vi "Update Messages Access Scope.vi"(8 "error in (no error)":errorcluster, 9 "scope":T1(ring)=enum."private", 10 "message parameters":T2[](array[typedef]), 11 "library in":refnum<vi>) -> (0 "error out":errorcluster, 3 "library out":refnum<vi>)   [LabVIEW 2019, in "gRPC Template Creation Utility.lvlib"]
uses:
  gRPC Template Creation Utility.lvlib
  TypeDefs/Message Metadata (Scripting).ctl
  TypeDefs/Message Element Metadata (Scripting).ctl
  TypeDefs/Message Element Type.ctl
  Oneof API/OneOf Constants/OneOfConstantsEnum.ctl
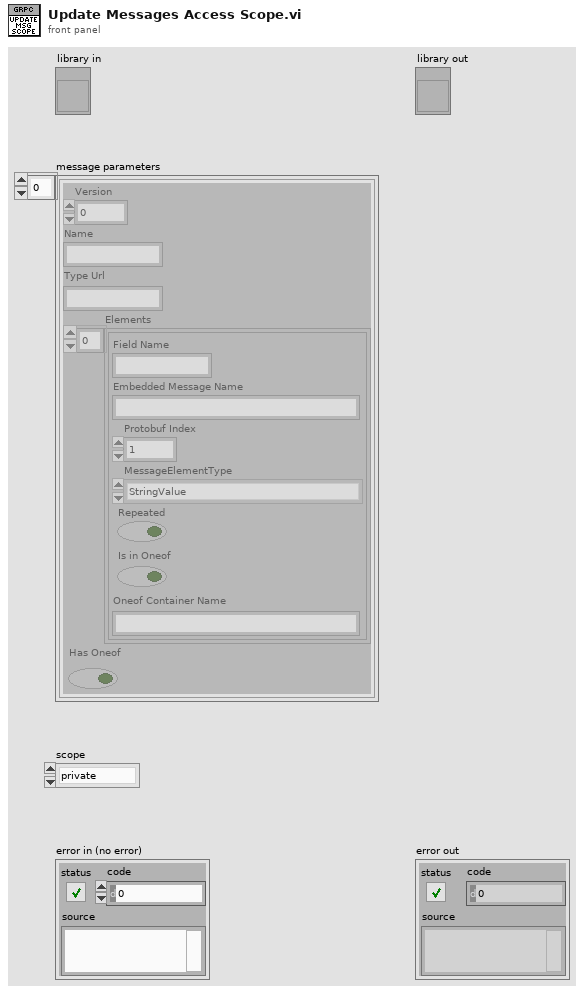
[diagram p1: front panel]
types:
  T1 = enum32{"invalid scope", "public", "private", "protected", "community"}
  T2 = typedef "gRPC Template Creation Utility.lvlib/Message Metadata (Scripting).ctl" = cluster{"Version":i32, "Name":string, "Type Url":string, "Elements":T3[], "Has Oneof":bool}
  T3 = typedef "gRPC Template Creation Utility.lvlib/Message Element Metadata (Scripting).ctl" = cluster{"Field Name":string, "Embedded Message Name":string, "Protobuf Index":i32, "MessageElementType":T4, "Repeated":bool, "Is in Oneof":bool, "Oneof Container Name":string}
  T4 = typedef "gRPC Template Creation Utility.lvlib/Message Element Type.ctl" = enum32{"Int32Value", "FloatValue", "DoubleValue", "BoolValue", "StringValue", "MessageValue", "Int64Value", "UInt32Value", "UInt64Value", "EnumValue", "Bytes", "Fixed64", "Fixed32", "SFixed64", "SFixed32", "SInt64", "SInt32"}
  T5 = typedef "gRPC Template Creation Utility.lvlib/OneOfConstantsEnum.ctl" = enum16{"FlatToRichVIPrefix", "RichToFlatVIPrefix", "FlatTypeDefSuffix"}
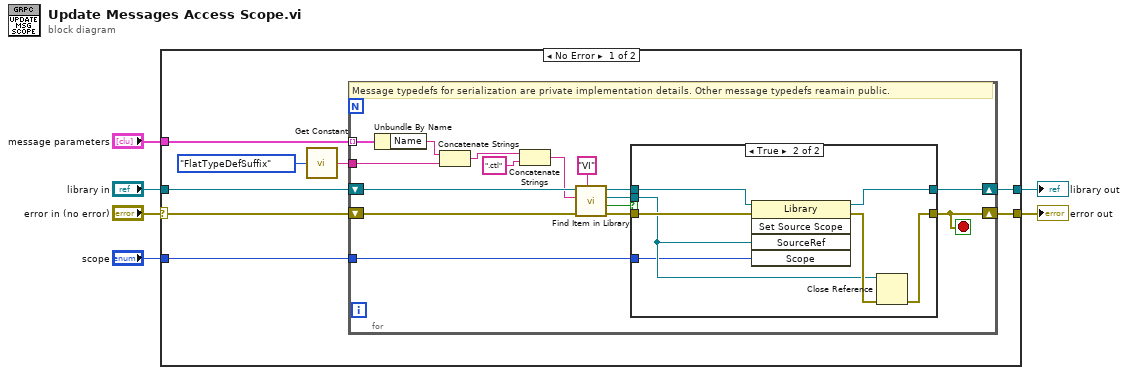
[diagram p0: block diagram]
diagram:
  n1 = case shown="No Error" "error in (no error)" {
    selector: "error in (no error)" -> [w10 w40]
    tunnel: "message parameters" -> [w14 _]
    tunnel: [w13 w41] -> w5
    tunnel: [w12 w40] -> w4
    tunnel: "library in" -> [w11 w41]
    tunnel: "scope" -> [w9 _]
    frame No Error {
      n2 = call "Get Constant.vi"("Selection"=OneOfConstantsEnum."FlatTypeDefSuffix") -> ("String"=w8:string)
      n3 = for {
        shift-right: [w18] -> w13
        shift-left: w11 -> [w26]
        shift-right: [w17] -> w12
        shift-left: w10 -> [w19]
        tunnel: w14 -> [w30] mode=indexing
        tunnel: w9 -> [w16]
        tunnel: w8 -> [w15]
        stop <- w17 stop-if-true
        # "Message typedefs for serialization are private implementation details. Other message typedefs reamain public."
        n4 = Unbundle By Name(w30) -> ("Name"=w27:string)
        n5 = Concatenate Strings(w27, w15) -> (w28:string)
        n6 = Concatenate Strings(w28, ".ctl" ("string")) -> (w25:string)
        n7 = call "Find Item in Library.vi"("Item Type"="VI" ("Type"), "error in (no error)"=w19, "Item Name"=w25, "Library item in"=w26) -> ("error out"=w20:errorcluster, "Found?"=w22:bool, "Project Item (Library Item)"=w23:refnum<vi>, "Library item out"=w21:refnum<vi>)  [unwired: 4 in]
        n8 = case shown="True" w22 {
          tunnel: w20 -> [w31 w37]
          tunnel: w23 -> [_ w34]
          tunnel: [w31 w35] -> w17
          tunnel: w21 -> [w32 w39]
          tunnel: [w32 w38] -> w18
          tunnel: w16 -> [_ w33]
          frame False {
          }
          frame True {
            n9 = invoke class="Library" method="Set Source Scope"(reference=w39, error in=w37, "SourceRef"=w34, "Scope"=w33) -> (reference out=w38:refnum<vi>, error out=w36:errorcluster)  [unwired: 1 in, 3 out]
            n10 = Close Reference(reference=w34, error in (no error)=w36) -> (error out=w35:errorcluster)
          }
        }
      }
    }
    frame Error {
    }
  }
  "library out" <- w5
  "error out" <- w4
